vi "TEST - String to 1D Array.vi"(8 "error in (no error)":errorcluster) -> (0 "error out":errorcluster, 2 "pass":bool)   [LabVIEW 2020, in "test_openg_string.lvlib"]
uses:
  test_openg_string.lvlib
  source/library/openg_string.lvlib
panel:
  out "Failures":T1(array[cluster])
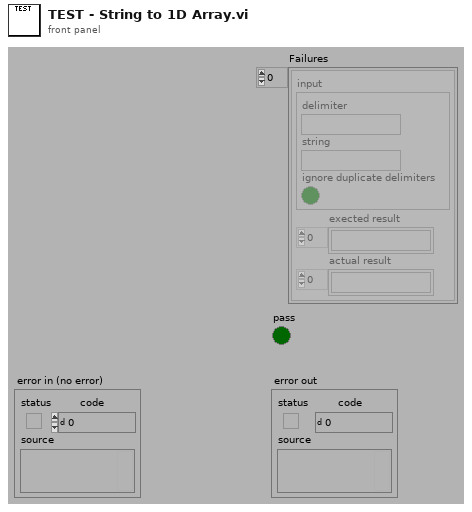
[diagram p1: front panel]
types:
  T1 = cluster{"input":cluster{"delimiter":string, "string":string, "ignore duplicate delimiters":bool}, "exected result":string[], "actual result":string[]}[]
  T2 = cluster{"input":cluster{"delimiter":string, "string":string, "ignore duplicate delimiters":bool}, "exected result":string[], "actual result":string[]}
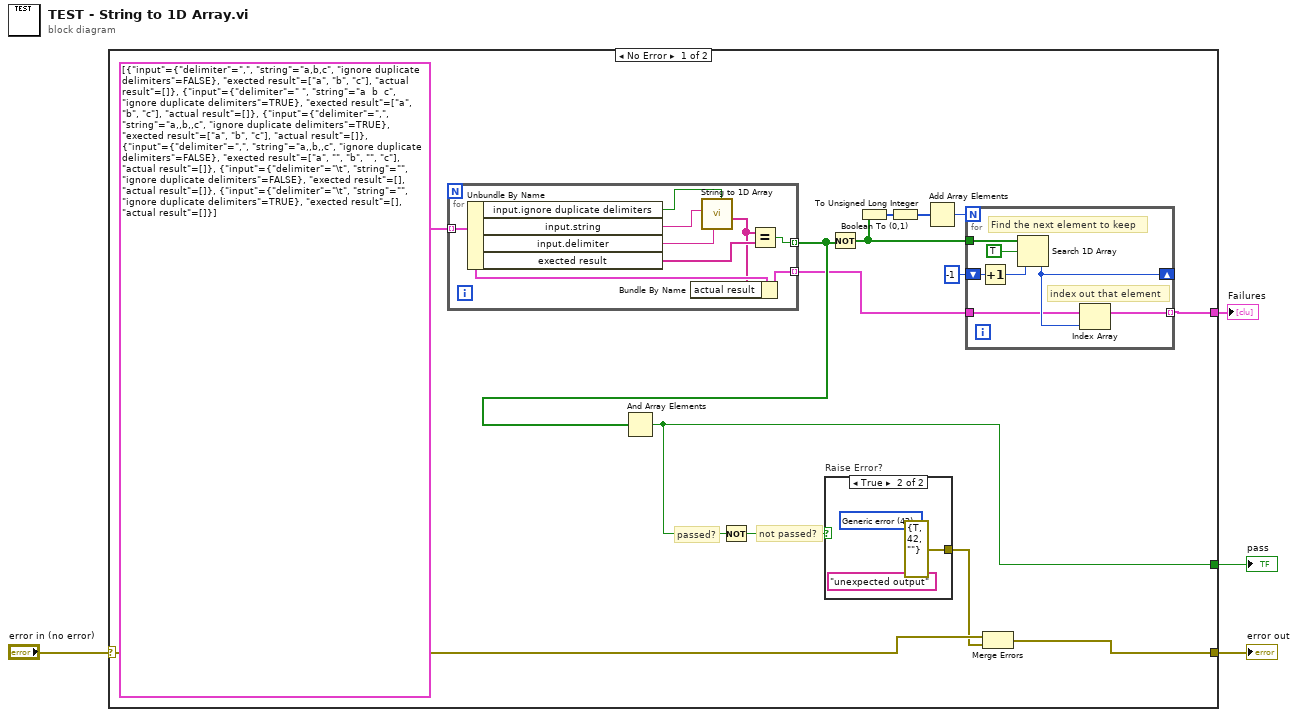
[diagram p0: block diagram]
diagram:
  n1 = case shown="No Error" "error in (no error)" {
    selector: "error in (no error)" -> [w18 w35]
    tunnel: [w13 _] -> w4
    tunnel: [w17 w35] -> w2
    tunnel: [w5 _] -> w1
    frame No Error {
      # "not passed?"
      # "passed?"
      n2 = for {
        tunnel: T1 [{"input"={"delimiter"=",", "string"="a,b,c", "ignore duplicate delimiters"=FALSE}, "exected result"=["a", "b", "c"], "actual result"=[]}, {"input"={"delimiter"=" ", "string"="a  b  c", "ignore duplicate delimiters"=TRUE}, "exected result"=["a", "b", "c"], "actual result"=[]}, {"input"={"delimiter"=",", "string"="a,,b,,c", "ignore duplicate delimiters"=TRUE}, "exected result"=["a", "b", "c"], "actual result"=[]}, {"input"={"delimiter"=",", "string"="a,,b,,c", "ignore duplicate delimiters"=FALSE}, "exected result"=["a", "", "b", "", "c"], "actual result"=[]}, {"input"={"delimiter"="\t", "string"="", "ignore duplicate delimiters"=FALSE}, "exected result"=[], "actual result"=[]}, {"input"={"delimiter"="\t", "string"="", "ignore duplicate delimiters"=TRUE}, "exected result"=[], "actual result"=[]}] -> [w30] mode=indexing
        tunnel: [w33] -> w7 mode=indexing
        tunnel: [w31] -> w6 mode=indexing
        n3 = Unbundle By Name(w30) -> ("input.ignore duplicate delimiters"=w26:bool, "input.string"=w29:string, "input.delimiter"=w27:string, "exected result"=w32:string[])
        n4 = call "String to 1D Array.vi"("ignore duplicate delimiters? (F=No)"=w26, "delimiter (Tab)"=w27, "string"=w29) -> ("Array of Strings"=w28:string[])  [unwired: 8 in]
        n5 = Bundle By Name(cluster=w30, "actual result"=w28) -> (w31:T2)
        n6 = Equal?(x=w28, y=w32) -> (x = y?=w33:bool)
      }
      n7 = And Array Elements(Boolean array=w7) -> (logical AND=w13:bool)
      n8 = Not(x=w13) -> (.not. x?=w15:bool)
      n9 = case "Raise Error?" shown="True" w15 {
        tunnel: [_ errorcluster {"status"=TRUE, "code"=42, "source"=""} ("error out")] -> w16
        frame False {
        }
        frame True {
          (unwired) 42 items=["No error", "Argument error", "Memory is full", "Out of zone", "End of file", "File already open", "Generic file I/O error", "File not found", "File permission error", "Disk is full", "Duplicate path", "Too many files open", "System feature not enabled", "Resource file not found", "Cannot add resource", "Resource not found", "Image not found", "Image memory error", "Pen does not exist", "Config type invalid", "Config token not found", "Config parse error", "Config memory error", "Bad external code format", "Bad external code offset", "External code not present", "Null window", "Destroy window error", "Null menu", "Print aborted", "Bad print record", "Print driver error", "Windows error during printing", "Memory error during printing", "Print dialog error", "Generic print error", "Invalid device refnum", "Device not found", "Device parameter error", "Device unit error", "Cannot open device", "Device call aborted", "Generic error", "Cancelled by user", "Object ID too low", "Object ID too high", "Object not in heap", "Unknown heap", "Unknown object (invalid DefProc)", "Unknown object (DefProc not in table)", "Message out of range", "Invalid (null) method", "Unknown message", "Manager call not supported", "Bad address", "Network operation in progress", "Network operation timed out", "Connection is busy", "Network attribute not supported", "Network error", "Address in use", "System out of memory", "Connection aborted", "Connection refused", "Not connected", "Already connected", "Connection closed", "Initialization error (interapplication manager)", "Bad occurrence", "Wait on unbound occurrence handler", "Occurrence queue overflow", "Datalog type conflict", "Unused", "Unrecognized type (interapplication manager)", "Memory corrupt", "Failed to make temporary DLL", "Old CIN version", "Drag socket not found", "Failed to load drop-object", "Failed to register OLE object", "Failed to release OLE object", "Format specifier type mismatch", "Unknown format specifier", "Too few format specifiers", "Too many format specifiers", "Scan failed", "Newer CIN version", "Error converting to variant", "Runtime menu error", "Password tampered", "Variant attribute not found", "Incompatible variant data type", "Event data is not available", "Event Store is not present", "Occurrence is not found", "Event Queue is not created", "Event info is not available", "Refnum passed is NULL", "Error retrieving Class GUID", "Error retrieving CoClass GUID", "Error retrieving TypeLib GUID.", "Bad built application magic bytes.", "Specific driver is different from the specific driver associated with the Logical Name.", "There is no session opened to the class driver.", "Max Error", "MAX - Error with config objects", "MAX - Error loading configuration", "MAX - Group not supported"]
          (unwired) "unexpected output" ("String to Prepend to source (\"\")")
        }
      }
      n10 = Not(x=w7) -> (.not. x?=w9:bool[])
      n11 = Boolean To (0,1)(Boolean=w9) -> (0, 1=w10:i16[])
      n12 = To Unsigned Long Integer(number=w10) -> (unsigned 32bit integer=w8:u32[])
      n13 = Add Array Elements(numeric array=w8) -> (sum=w11:u32)
      n14 = for {
        N: w11 -> [_]
        tunnel: w6 -> [w21]
        tunnel: w9 -> [w25]
        shift-right: [w22] -> _
        shift-left: -1 ("start index (0)") -> [w23]
        tunnel: [w20] -> w5 mode=indexing
        # "index out that element"
        # "Find the next element to keep"
        n15 = Increment(x=w23) -> (x+1=w19:i32)
        n16 = Search 1D Array(1D array=w25, element=TRUE, start index (0)=w19) -> (index of element=w22:i32)
        n17 = Index Array(array=w21, index=w22) -> (element=w20:T2)
      }
      n18 = Merge Errors(w18, w16) -> (w17:errorcluster)
    }
    frame Error {
    }
  }
  "pass" <- w4
  "error out" <- w2
  "Failures" <- w1
